vi "Report - Generate Report.vi"(8 "error in":errorcluster, 11 "Fileid":string) -> (0 "error out":errorcluster)   [LabVIEW 2019]
uses:
  Controls/Report - State.ctl
  Controls/Report - Data Structure.ctl
  <vilib>/httpClient/ClientHandle.ctl
  Controls/FGV States.ctl
  Controls/eFGV States.ctl
  Controls/JSON - Fileid.ctl
  Controls/JSON - Report.ctl
  <vilib>/Utility/sysdir.llb/System Directory Type.ctl
  <vilib>/httpClient/POSTBuffer.vi
  <userlib>/_OpenG.lib/array/array.llb/Remove Duplicates from 1D Array (String)__ogtk.vi
  <userlib>/_OpenG.lib/array/array.llb/Delete Elements from 1D Array (String)__ogtk.vi
  <vilib>/Utility/config.llb/Read Key (String).vi
  <vilib>/httpClient/LabVIEWHTTPClient.lvlib
  <vilib>/Utility/config.llb/NI_LVConfig.lvlib
panel:
  in  "Plot":bool
  out "Current stage":T1
  in  "Back":bool
  in  "Forward":bool
  in  "Pages":u32
  out "Total":u32
  out "data":T2(array[cluster])
  in  "Cancel":bool
  in  "Generate":bool
  in  "Search":string
  in  "Listbox":i32(listbox)=-1 caption="Select File to Export"
  # "of"
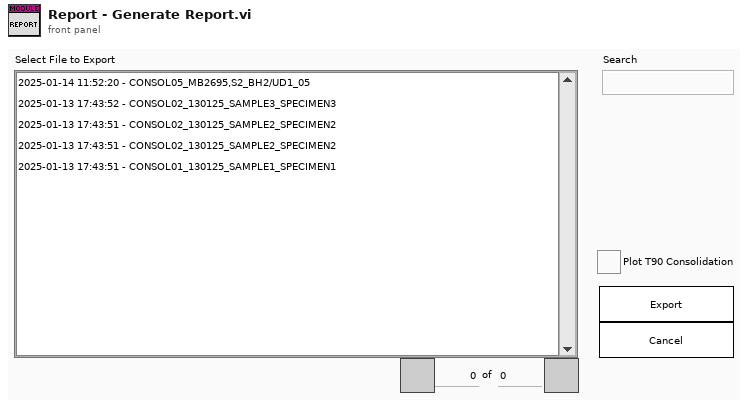
[diagram p1: front panel]
types:
  T1 = typedef "Report - State.ctl" = enum16{"Init", "Get File List", "Get Station Name", "Parse File List", "Idle", "Prepare to Generate", "Get Report", "Parse Report", "Get Data", "View T90", "Parse Data", "Convert to Excel", "Clean Up", "Close"}
  T2 = cluster{"id":string, "created_date":string, "testname":string, "jobno":string, "jobdesc":string, "sampleid":string, "date":string, "specimentno":string, "depth":string, "height":string, "diameter":string, "weight":string, "done":string}[]
  T3 = typedef "eFGV States.ctl" = enum16{"Init", "Read", "Write", "Exit"}
  T4 = typedef "FGV States.ctl" = enum16{"Read", "Write"}
  T5 = typedef "Report - Data Structure.ctl" = cluster{"API Ref":T6, "FileList":string[][], "Fileid":string, "testname":string[], "testtype":string[], "tdms":refnum<k34>, "TDMS Path":path, "tdms_path":string, "excel_path":string, "Excel Path":path, "List Name":string[], "Station Name":string[], "Plot":bool, "Tangent Point":string}
  T6 = typedef "LabVIEWHTTPClient.lvlib/ClientHandle.ctl" = refnum<k1>
  T7 = enum32{"Invalid", "Default", "Floating", "Floating/Auto-Hide", "Modal"}
  T8 = enum32{"Invalid", "Standard", "Closed", "Hidden", "Minimized", "Maximized"}
  T9 = typedef "JSON - Fileid.ctl" = cluster{"status":string, "data":cluster{"id":string, "created_date":string, "testname":string, "jobno":string, "jobdesc":string, "sampleid":string, "date":string, "specimentno":string, "depth":string, "height":string, "diameter":string, "weight":string, "done":string}[]}
  T10 = cluster{"status":string, "data":cluster{"id":string, "created_date":string, "filename":string, "stage":string, "testplan":string, "station":string, "status":string, "delete":string}[]}
  T11 = typedef "JSON - Report.ctl" = cluster{"status":string, "data":cluster{"testname":string, "testtype":string}[]}
  T12 = enum16{"open", "open or create", "create or replace", "create", "open (read-only)"}
  T13 = cluster{"id":string, "created_date":string, "filename":string, "stage":string, "testplan":string, "station":string, "status":string, "delete":string}[]
  T14 = cluster{"id":string, "created_date":string, "filename":string, "stage":string, "testplan":string, "station":string, "status":string, "delete":string}
  T15 = typedef "eventvkey.ctl" = enum16{"ASCII", "Enter", "Return", "Shift", "Ctrl", "Alt", "Cmd", "Opt", "Caps", "NumLock", "Clear", "Break", "Up", "Down", "Left", "Right", "Insert", "Delete", "Home", "End", "PageUp", "PageDown", "Escape", "Help", "Pause", "ScrollLock", "F1", "F2", "F3", "F4", "F5", "F6", "F7", "F8", "F9", "F10", "F11", "F12", "F13", "F14", "F15", "F16", "F17", "F18", "F19", "F20", "F21", "F22", "F23", "F24", "Play", "VolumeUp", "VolumeDown", "Mute", "Two Byte Char"}
  T16 = typedef "System Directory Type.ctl" = i32
  T17 = typedef "NI_LVConfig.lvlib/Config Data RefNum.ctl" = refnum<k1>
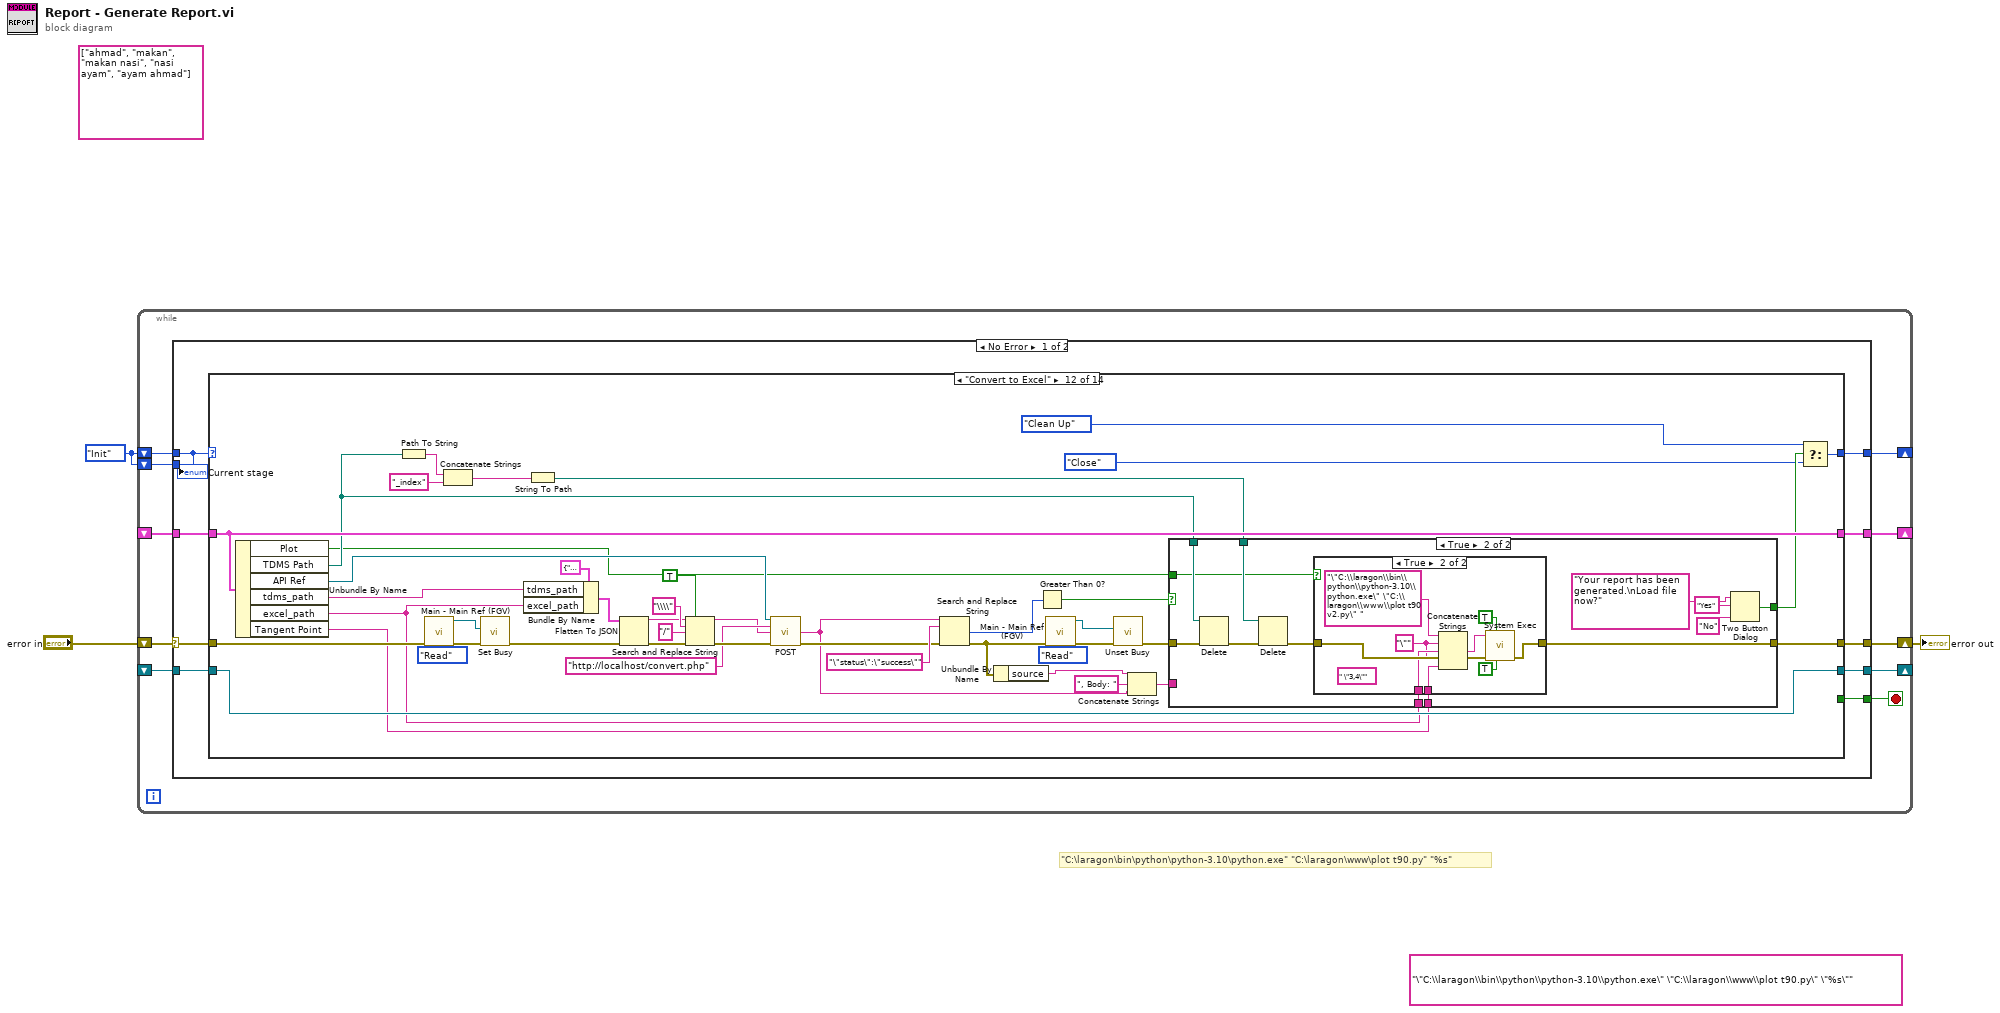
[diagram p0: block diagram]
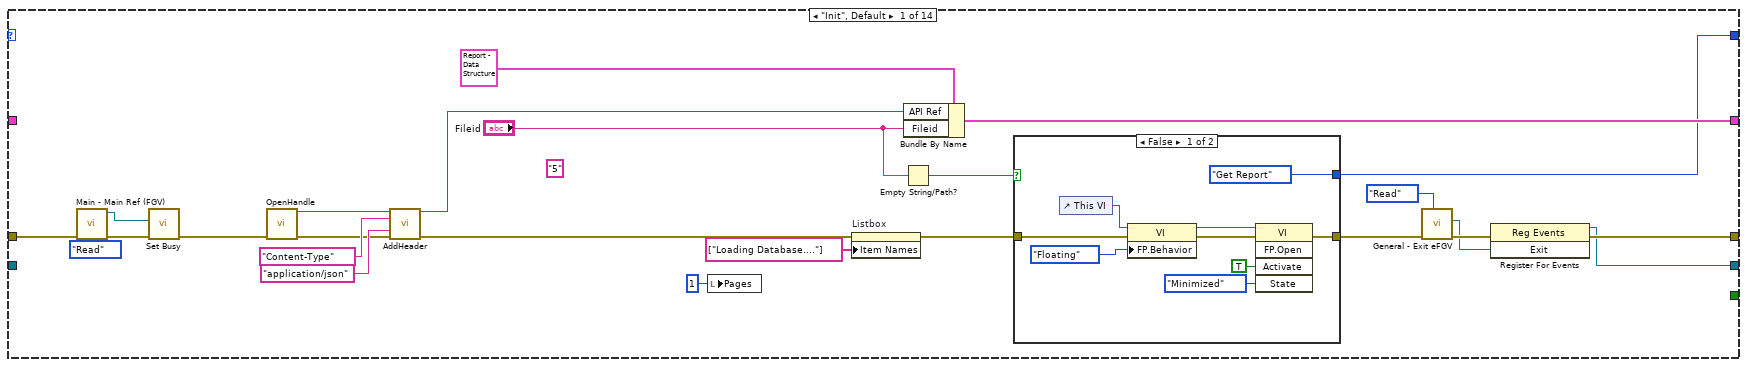
[diagram p2: hidden frame]
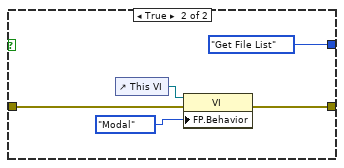
[diagram p3: hidden frame]
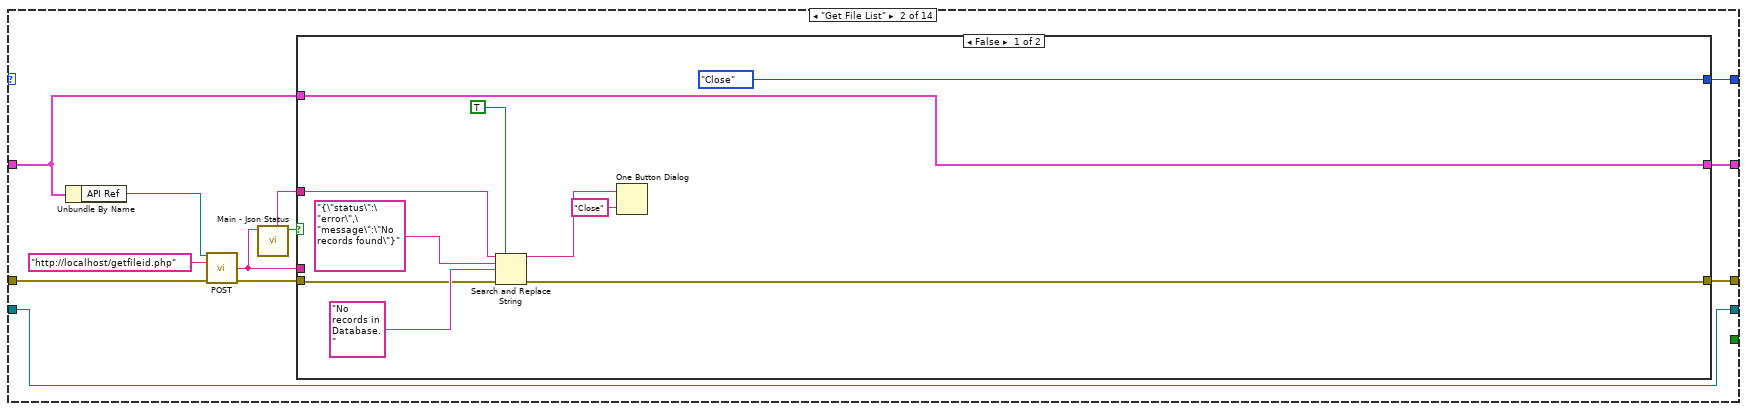
[diagram p4: hidden frame]
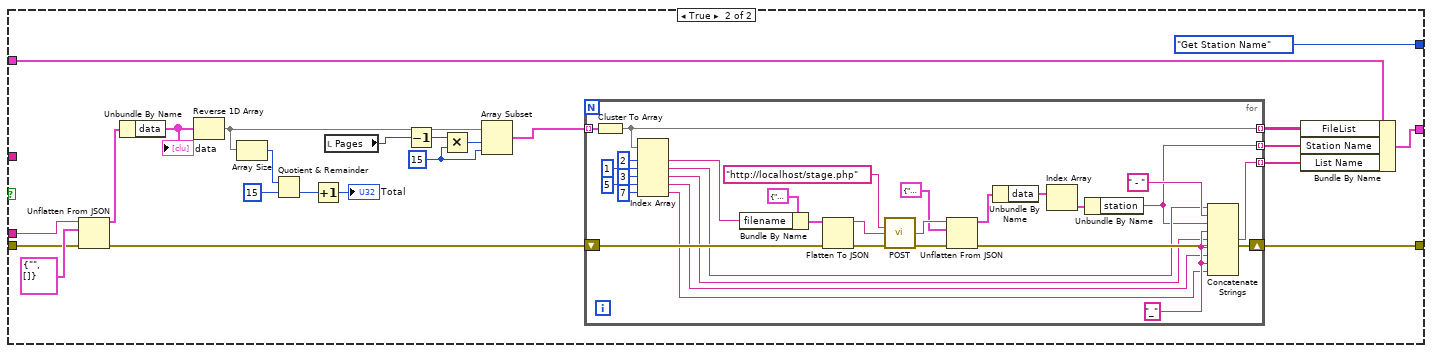
[diagram p5: hidden frame]
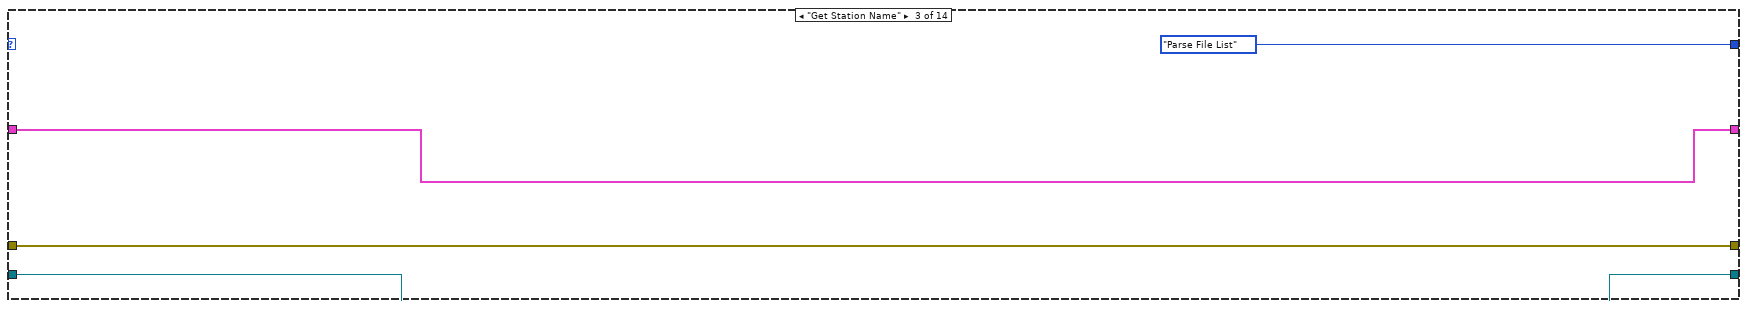
[diagram p6: hidden frame]
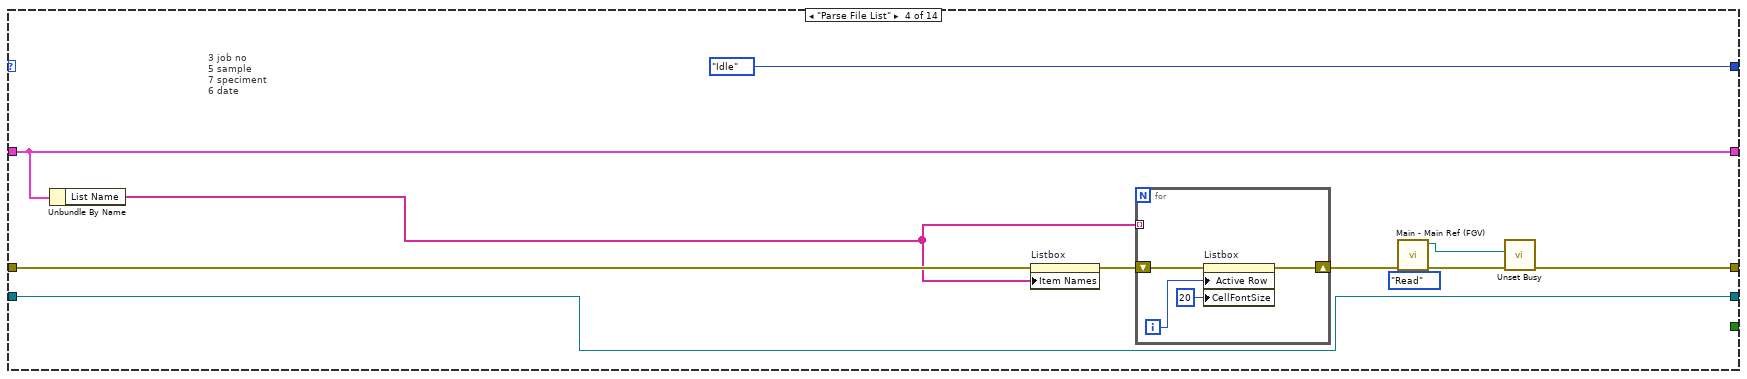
[diagram p7: hidden frame]
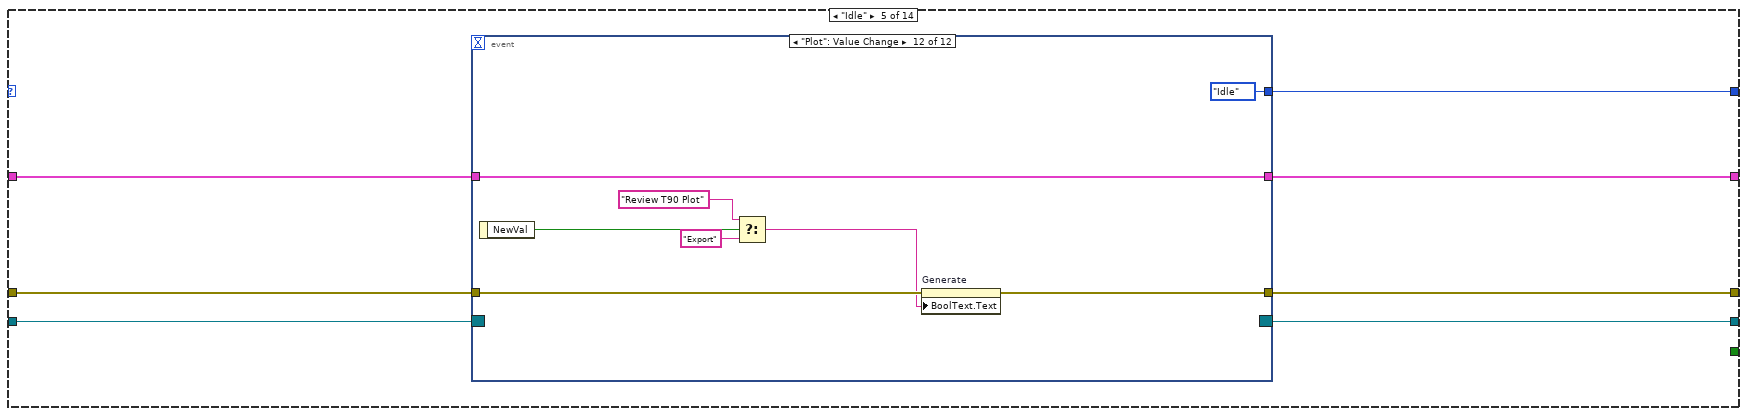
[diagram p8: hidden frame]
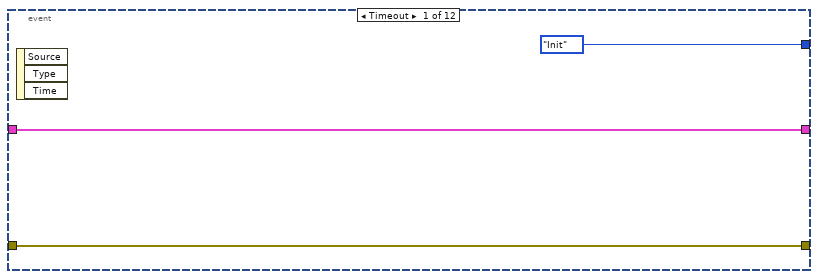
[diagram p9: hidden frame]
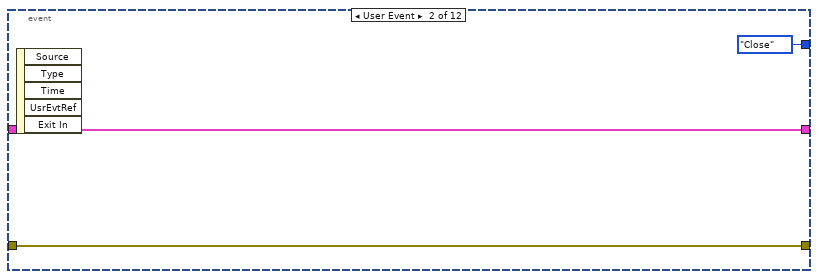
[diagram p10: hidden frame]
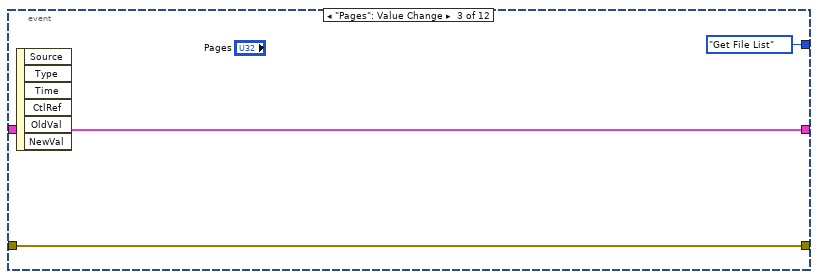
[diagram p11: hidden frame]
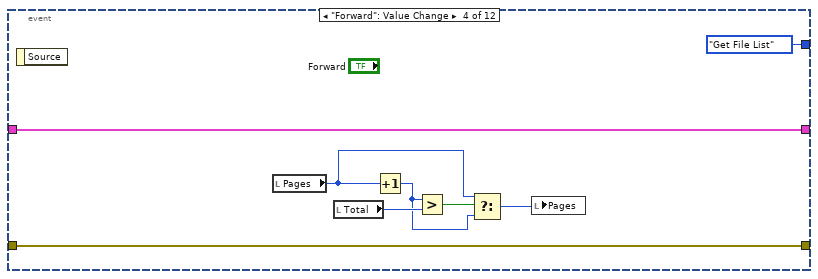
[diagram p12: hidden frame]
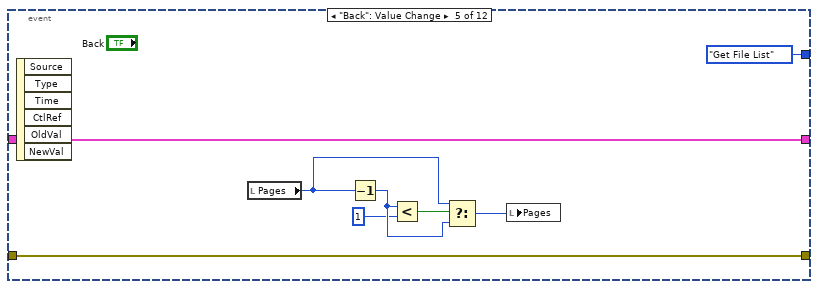
[diagram p13: hidden frame]
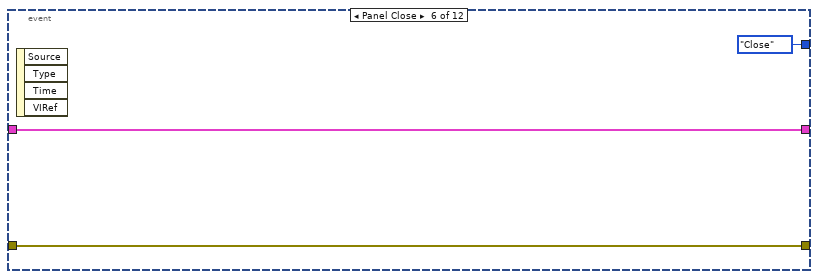
[diagram p14: hidden frame]
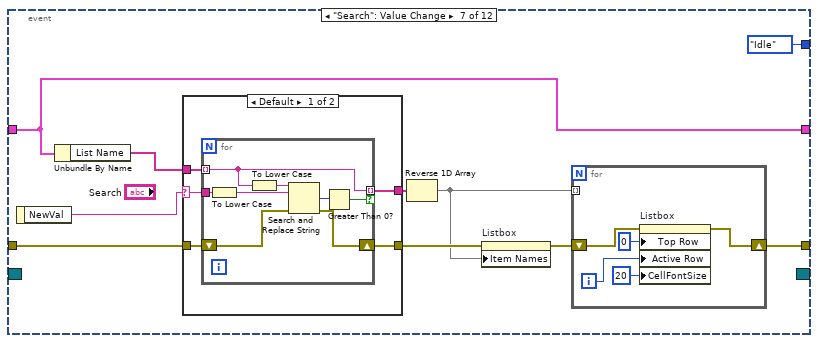
[diagram p15: hidden frame]
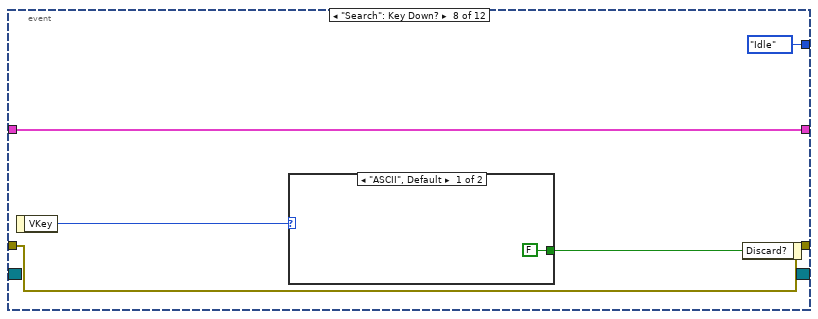
[diagram p17: hidden frame]
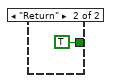
[diagram p18: hidden frame]
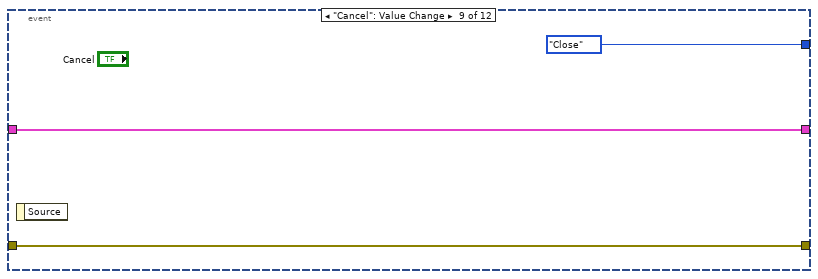
[diagram p19: hidden frame]
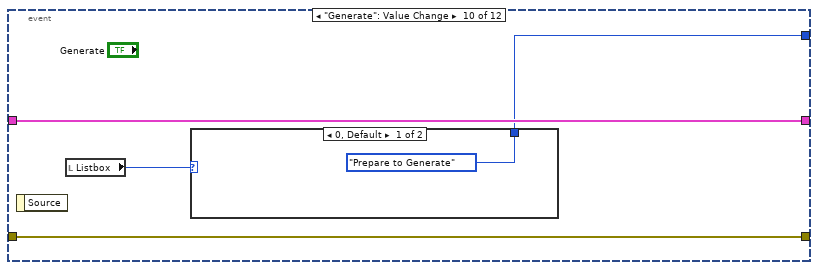
[diagram p20: hidden frame]
diagram:
  (unwired) "\"C:\\laragon\\bin\\python\\python-3.10\\python.exe\" \"C:\\laragon\\www\\plot t90.py\" \"%s\"" ("command line")
  w1 = Report_-_State."Init"
  (unwired) string[] ["ahmad", "makan", "makan nasi", "nasi ayam", "ayam ahmad"]
  # "\"C:\\laragon\\bin\\python\\python-3.10\\python.exe\" \"C:\\laragon\\www\\plot t90.py\" \"%s\""
  n1 = while {
    shift-right: [w10] -> w2
    shift-left: "error in" -> [w13]
    shift-right: [w11] -> _
    shift-left: w1 -> [w12]
    shift-right: [w9] -> _
    shift-left: _ -> [w8]
    shift-left: w1 -> [w6]
    shift-right: [w5] -> _
    shift-left: _ -> [w4]
    stop <- w7 stop-if-true
    n2 = case shown="No Error" w13 {
      selector: w13 -> [w20 w547]
      tunnel: w12 -> [w22 _]
      tunnel: [w21 Report_-_State."Close"] -> w11
      tunnel: [w19 w544] -> w10
      tunnel: [w18 w545] -> w9
      tunnel: w8 -> [w17 w545]
      tunnel: [w16 _] -> w7
      tunnel: w6 -> [_ w538]
      tunnel: [w15 w534] -> w5
      tunnel: w4 -> [w14 w534]
      frame No Error {
        n3 = case shown="\"Convert to Excel\"" w22 {
          tunnel: [w40 w71 Report_-_State."Parse File List" Report_-_State."Idle" w159 Report_-_State."Get Report" w285 Report_-_State."Get Data" w344 Report_-_State."Parse Data" w384 w429 Report_-_State."Close" Report_-_State."Idle"] -> w21
          tunnel: w20 -> [w35 w72 w139 w149 w161 w268 w298 w331 w345 w372 w377 w425 w493 w530]
          tunnel: [w29 w69 w139 w143 w160 w282 w289 w328 w341 w371 w382 w433 w498 w522] -> w19
          tunnel: [w41 w66 w137 w147 w157 w273 w290 w327 w339 w367 w386 w432 w497 T5 {"API Ref"=refnum, "FileList"=[], "Fileid"="", "testname"=[], "testtype"=[], "tdms"=refnum, "TDMS Path"=path "", "tdms_path"="", "excel_path"="", "Excel Path"=path "", "List Name"=[], "Station Name"=[], "Plot"=FALSE, "Tangent Point"=""}] -> w18
          tunnel: w17 -> [_ w67 w137 w147 w158 w272 w292 w330 w338 w366 w389 w432 w497 w529]
          tunnel: [_ _ _ _ _ _ _ _ _ _ _ _ _ TRUE] -> w16
          tunnel: [w27 w62 w136 w140 w155 w265 w284 w323 w340 w373 w374 w413 w484 w521] -> w15
          tunnel: w14 -> [_ w62 w136 w140 w156 w265 w284 w323 w340 w373 w374 w413 w484 w521]
          frame "Init", Default {
            (unwired) "5"
            n4 = call "Main - Main Ref (FGV).vi"("Action"=FGV_States."Read", "error in"=w35) -> ("error out"=w36:errorcluster, "This VI out"=w34:refnum<vi>)  [unwired: 8 in]
            n5 = call <vilib>:"Set Busy.vi"("error in (no error)"=w36, "VI reference (current VI)"=w34) -> ("error out"=w38:errorcluster)  [unwired: 8 in, 1 out]
            n6 = call <vilib>:"OpenHandle.vi"("error in (no error)"=w38) -> ("client handle out"=w45:T6, "error out"=w44:errorcluster)  [unwired: 13 in]
            n7 = call <vilib>:"AddHeader.vi"("client handle"=w45, "header"="Content-Type", "value"="application/json", "error in (no error)"=w44) -> ("client handle out"=w42:T6, "error out"=w26:errorcluster)  [unwired: 10 in]
            n8 = local write "Pages"(u32 1 ("Pages")) -> ()
            n9 = property on="Listbox" class="LstBox (strict)"(error in=w26, "Item Names"=string[] ["Loading Database...."]) -> (error out=w25:errorcluster)  [unwired: 1 in, 1 out]
            n10 = Empty String/Path?(string/path="Fileid") -> (empty?=w39:bool)
            n11 = Bundle By Name(cluster=T5 {"API Ref"=refnum, "FileList"=[], "Fileid"="", "testname"=[], "testtype"=[], "tdms"=refnum, "TDMS Path"=path "", "tdms_path"="", "excel_path"="", "Excel Path"=path "", "List Name"=[], "Station Name"=[], "Plot"=FALSE, "Tangent Point"=""}, "API Ref"=w42, "Fileid"="Fileid") -> (w41:T5)
            n12 = case shown="False" w39 {
              tunnel: [Report_-_State."Get Report" ("f") Report_-_State."Get File List" ("f")] -> w40
              tunnel: w25 -> [w52 w58]
              tunnel: [w50 w57] -> w32
              frame False {
                n13 = control-ref of="This VI"() -> (w49:refnum<vi>)
                n14 = property class="VI"(reference=w49, error in=w52, "FP.Behavior"=T7."Floating" ("Front Panel Window:Behavior")) -> (reference out=w48:refnum<vi>, error out=w51:errorcluster)
                n15 = invoke class="VI" method="FP.Open"(reference=w48, error in=w51, "Activate"=TRUE ("Activate?"), "State"=T8."Minimized") -> (error out=w50:errorcluster)  [unwired: 1 in, 4 out]
              }
              frame True {
                n16 = control-ref of="This VI"() -> (w60:refnum<vi>)
                n17 = property class="VI"(reference=w60, error in=w58, "FP.Behavior"=T7."Modal" ("Front Panel Window:Behavior")) -> (error out=w57:errorcluster)  [unwired: 1 out]
              }
            }
            n18 = call "General - Exit eFGV.vi"("eFGV States"=eFGV_States."Read", "error in (no error)"=w32) -> ("error out"=w31:errorcluster, "Exit"=w28:refnum<user-event>)  [unwired: 7 in, 1 out]
            n19 = register-events(error in=w31, w28) -> (reference out=w27:refnum<event-registration>, error out=w29:errorcluster)  [unwired: 1 in]
          }
          frame "Get File List" {
            n20 = Unbundle By Name(w67) -> ("API Ref"=w68:T6)
            n21 = call-poly <vilib>:"POST.vi"("client handle"=w68, "url"="http://localhost/getfileid.php", "error in (no error)"=w72) -> ("body"=w65:string, "error out"=w70:errorcluster)  [unwired: 9 in, 2 out]
            n22 = call "Main - Json Status.vi"("json"=w65) -> ("Success?"=w64:bool, "message"=w63:string)  [unwired: 9 in]
            n23 = case shown="False" w64 {
              tunnel: [Report_-_State."Close" Report_-_State."Get Station Name"] -> w71
              tunnel: w70 -> [w74 w104]
              tunnel: [w75 w97] -> w69
              tunnel: w65 -> [_ w103]
              tunnel: w67 -> [w82 w100]
              tunnel: [w82 w98] -> w66
              tunnel: w63 -> [w77 _]
              frame False {
                n24 = Search and Replace String(replace all?=TRUE ("replace all? (F)"), input string=w77, search string="{\"status\":\"error\",\"message\":\"No records found\"}", replace string="No records in Database." ("replace string (\"\")"), error in=w74) -> (result string=w78:string, error out=w75:errorcluster)  [unwired: 3 in, 2 out]
                n25 = One Button Dialog(message=w78, button name ("OK")="Close") -> ()  [unwired: 1 out]
              }
              frame True {
                w90 = 15 ("length")
                n26 = Unflatten From JSON(JSON string=w103, type and defaults=T9 {"status"="", "data"=[]}, error in (no error)=w104) -> (value=w101:T9, error out=w85:errorcluster)  [unwired: 4 in]
                n27 = Unbundle By Name(w101) -> ("data"=w102:T2)
                "data" <- w102
                n28 = Reverse 1D Array(array=w102) -> (reversed array=w89:T2)
                n29 = Array Size(array=w89) -> (size(s)=w93:i32)
                n30 = Quotient & Remainder(x=w93, y=15) -> (floor(x/y)=w94:i32)  [unwired: 1 out]
                n31 = Increment(x=w94) -> (x+1=→"Total":i32)
                n32 = local read "Pages"() -> (w86:u32)
                n33 = Decrement(x=w86) -> (x-1=w87:u32)
                n34 = Multiply(x=w87, y=w90) -> (x*y=w91:u32)
                n35 = Array Subset(array=w89, index=w91, length=w90) -> (w88:T2)
                n36 = for {
                  tunnel: w88 -> [w135] mode=indexing
                  tunnel: [w134] -> w99 mode=indexing
                  shift-right: [w114] -> w97
                  shift-left: w85 -> [w115]
                  tunnel: [w108] -> w95 mode=indexing
                  tunnel: [w107] -> w96 mode=indexing
                  w119 = "_" ("string")
                  n37 = Cluster To Array(cluster=w135) -> (array=w134:string[])
                  n38 = Index Array(array=w134, index #1=2 ("disabled index (col)"), index #2=1 ("index (col)"), index #3=3 ("index (col)"), index #4=5 ("index (col)"), index #5=7 ("index (col)")) -> (element #1=w113:string, element #2=w112:string, element #3=w111:string, element #4=w110:string, element #5=w109:string)
                  n39 = Bundle By Name(cluster=cluster{"action":string, "filename":string} {"action"="read", "filename"=""}, "filename"=w113) -> (w124:cluster{"action":string, "filename":string})
                  n40 = Flatten To JSON(anything=w124, error in (no error)=w115) -> (JSON string=w125:string, 11:w128:errorcluster)  [unwired: 1 in]
                  n41 = call-poly <vilib>:"POST.vi"("url"="http://localhost/stage.php", "buffer"=w125, "error in (no error)"=w128) -> ("body"=w126:string, "error out"=w127:errorcluster)  [unwired: 9 in, 2 out]
                  n42 = Unflatten From JSON(JSON string=w126, type and defaults=T10 {"status"="read", "data"=[]} ("Cluster"), error in (no error)=w127) -> (value=w123:T10, error out=w114:errorcluster)  [unwired: 4 in]
                  n43 = Unbundle By Name(w123) -> ("data"=w122:T13)
                  n44 = Index Array(array=w122) -> (element=w121:T14)  [unwired: 1 in]
                  n45 = Unbundle By Name(w121) -> ("station"=w107:string)
                  n46 = Concatenate Strings(w112, " - " ("string"), w107, w119, w111, w119, w110, w119, w109) -> (w108:string)
                }
                n47 = Bundle By Name(cluster=w100, "FileList"=w99, "Station Name"=w96, "List Name"=w95) -> (w98:T5)
              }
            }
          }
          frame "Get Station Name" {
          }
          frame "Parse File List" {
            # "3 job no\n5 sample\n7 speciment\n6 date"
            n48 = Unbundle By Name(w147) -> ("List Name"=w141:string[])
            n49 = property on="Listbox" class="LstBox (strict)"(error in=w149, "Item Names"=w141) -> (error out=w148:errorcluster)  [unwired: 1 in, 1 out]
            n50 = for {
              shift-right: [w152] -> w145
              shift-left: w148 -> [w153]
              tunnel: w141 -> [_] mode=indexing
              i -> [w151]
              n51 = property on="Listbox" class="LstBox (strict)"(error in=w153, "Active Row"=w151, "CellFontSize"=u32 20 ("Active Row:Cell Font:Size")) -> (error out=w152:errorcluster)  [unwired: 1 in, 1 out]
            }
            n52 = call "Main - Main Ref (FGV).vi"("Action"=FGV_States."Read", "error in"=w145) -> ("error out"=w144:errorcluster, "This VI out"=w142:refnum<vi>)  [unwired: 8 in]
            n53 = call <vilib>:"Unset Busy.vi"("error in (no error)"=w144, "VI reference (current VI)"=w142) -> ("error out"=w143:errorcluster)  [unwired: 9 in]
          }
          frame "Idle" {
            n54 = event shown="[11] \"Plot\": Value Change" {
              selector: w156 -> [_ _ _ _ _ _ _ _ _ _ _ _]
              dyn-events: [_ _ _ _ _ _ _ _ _ _ _ _] -> w155
              timeout: _ -> [_ _ _ _ _ _ _ _ _ _ _ _]
              tunnel: w161 -> [w164 w167 w168 w176 w186 w187 w195 w220 w228 w232 w249 w260]
              tunnel: [w164 w167 w168 w176 w186 w187 w194 w220 w228 w232 w246 w261] -> w160
              tunnel: [Report_-_State."Init" Report_-_State."Close" ("f") Report_-_State."Get File List" ("f") Report_-_State."Get File List" ("f") Report_-_State."Get File List" ("f") Report_-_State."Close" Report_-_State."Idle" Report_-_State."Idle" ("f") Report_-_State."Close" w230 w237 Report_-_State."Idle" ("f")] -> w159
              tunnel: w158 -> [w162 w166 w170 w177 w185 w188 w192 w224 w229 w233 w252 w263]
              tunnel: [w162 w166 w170 w177 w185 w188 w192 w224 w229 w233 w252 w263] -> w157
              event Timeout {
                n55 = event-data() -> ()  [unwired: 1 in, 3 out]
              }
              event User Event {
                n56 = event-data() -> ()  [unwired: 1 in, 5 out]
              }
              event "Pages": Value Change {
                n57 = event-data() -> ()  [unwired: 1 in, 6 out]
              }
              event "Forward": Value Change {
                n58 = event-data() -> ()  [unwired: 1 in, 1 out]
                n59 = local read "Pages"() -> (w173:u32)
                n60 = local read "Total"() -> (w175:u32)
                n61 = Increment(x=w173) -> (x+1=w172:u32)
                n62 = Greater?(x=w172, y=w175) -> (0:w174:bool)
                n63 = Select(t=w173, s=w174, f=w172) -> (s? t:f=w171:u32)
                n64 = local write "Pages"(w171) -> ()
              }
              event "Back": Value Change {
                n65 = event-data() -> ()  [unwired: 1 in, 6 out]
                n66 = local read "Pages"() -> (w182:u32)
                n67 = Decrement(x=w182) -> (x-1=w181:u32)
                n68 = Less?(x=w181, y=u32 1) -> (x < y?=w183:bool)
                n69 = Select(t=w182, s=w183, f=w181) -> (s? t:f=w180:u32)
                n70 = local write "Pages"(w180) -> ()
              }
              event Panel Close {
                n71 = event-data() -> ()  [unwired: 1 in, 4 out]
              }
              event "Search": Value Change {
                n72 = event-data() -> ("NewVal"=w193:string)  [unwired: 1 in]
                n73 = Unbundle By Name(w192) -> ("List Name"=w190:string[])
                n74 = case shown="Default" w193 {
                  selector: w193 -> [w205 _]
                  tunnel: w190 -> [w209 w219]
                  tunnel: w195 -> [w208 w218]
                  tunnel: [w207 w218] -> w198
                  tunnel: [w206 w219] -> w196
                  frame Default {
                    n75 = for {
                      tunnel: w205 -> [w217]
                      tunnel: [w214] -> w206 mode=indexing if=w215
                      tunnel: w209 -> [w214] mode=indexing
                      shift-right: [w212] -> w207
                      shift-left: w208 -> [w213]
                      n76 = To Lower Case(string=w217) -> (all lower case string=w211:string)
                      n77 = To Lower Case(string=w214) -> (all lower case string=w210:string)
                      n78 = Search and Replace String(input string=w210, search string=w211, error in=w213) -> (number of replacements=w216:i32, error out=w212:errorcluster)  [unwired: 5 in, 2 out]
                      n79 = Greater Than 0?(x=w216) -> (x > 0?=w215:bool)
                    }
                  }
                  frame "" {
                  }
                }
                n80 = Reverse 1D Array(array=w196) -> (reversed array=w191:string[])
                n81 = property on="Listbox" class="LstBox (strict)"(error in=w198, "Item Names"=w191) -> (error out=w197:errorcluster)  [unwired: 1 in, 1 out]
                n82 = for {
                  shift-right: [w202] -> w194
                  shift-left: w197 -> [w203]
                  tunnel: w191 -> [_] mode=indexing
                  i -> [w201]
                  n83 = property on="Listbox" class="LstBox (strict)"(error in=w203, "Top Row"=0, "Active Row"=w201, "CellFontSize"=u32 20 ("Active Row:Cell Font:Size")) -> (error out=w202:errorcluster)  [unwired: 1 in, 1 out]
                }
              }
              event "Search": Key Down? {
                n84 = event-data() -> ("VKey"=w222:T15)  [unwired: 1 in]
                n85 = case shown="\"ASCII\", Default" w222 {
                  tunnel: [FALSE TRUE] -> w221
                  frame "ASCII", Default {
                  }
                  frame "Return" {
                  }
                }
                n86 = event-data("Discard?"=w221) -> ()  [unwired: 1 in, 1 out]
              }
              event "Cancel": Value Change {
                n87 = event-data() -> ()  [unwired: 1 in, 1 out]
              }
              event "Generate": Value Change {
                n88 = event-data() -> ()  [unwired: 1 in, 1 out]
                n89 = local read "Listbox"() -> (w231:i32)
                n90 = case shown="0, Default" w231 {
                  tunnel: [Report_-_State."Prepare to Generate" Report_-_State."Idle"] -> w230
                  frame 0, Default {
                  }
                  frame -1 {
                    n91 = One Button Dialog(message="Please select a file") -> ()  [unwired: 1 in, 1 out]
                  }
                }
              }
              event "Listbox": Double Click {
                n92 = event-data() -> ("Row"=w247:i32)  [unwired: 1 in]
                n93 = property on="Listbox" class="LstBox (strict)"(error in=w249) -> (error out=w250:errorcluster, "Item Names"=w248:string[])  [unwired: 1 in, 1 out]
                n94 = Index Array(array=w248, index=w247) -> (element=w245:string)
                n95 = Format Into String(format string="Generate report %s?" ("message"), initial string="", error in=w250, w245) -> (resulting string=w242:string, error out=w246:errorcluster)
                n96 = Two Button Dialog(message=w242, 2:"Yes" ("T button name (\"OK\")")) -> (T button?=w238:bool)  [unwired: 1 in]
                n97 = local read "Listbox"() -> (w251:i32)
                n98 = case shown="0, Default" w251 {
                  tunnel: [Report_-_State."Prepare to Generate" Report_-_State."Idle"] -> w240
                  frame 0, Default {
                  }
                  frame -1 {
                    n99 = One Button Dialog(message="Please select a file") -> ()  [unwired: 1 in, 1 out]
                  }
                }
                n100 = Select(t=w240, s=w238, f=Report_-_State."Idle") -> (s? t:f=w237:T1)
              }
              event "Plot": Value Change {
                n101 = event-data() -> ("NewVal"=w258:bool)  [unwired: 1 in]
                n102 = Select(t="Review T90 Plot" ("Boolean Text.Text"), s=w258, f="Export") -> (s? t:f=w256:string)
                n103 = property on="Generate" class="Bool"(error in=w260, "BoolText.Text"=w256) -> (error out=w261:errorcluster)  [unwired: 1 in, 1 out]
              }
            }
          }
          frame "Prepare to Generate" {
            n104 = call "Main - Main Ref (FGV).vi"("Action"=FGV_States."Read", "error in"=w268) -> ("error out"=w269:errorcluster, "This VI out"=w267:refnum<vi>)  [unwired: 8 in]
            n105 = call <vilib>:"Set Busy.vi"("error in (no error)"=w269, "VI reference (current VI)"=w267) -> ("error out"=w271:errorcluster)  [unwired: 8 in, 1 out]
            n106 = property on="Listbox" class="LstBox (strict)"(error in=w271) -> (error out=w282:errorcluster, "Item Names"=w280:string[])  [unwired: 1 in, 1 out]
            n107 = Unbundle By Name(w272) -> ("FileList"=w279:string[][], "List Name"=w266:string[])
            n108 = Index Array(array=w279, index (col)=0 ("disabled index (col)")) -> (element=w276:string[])  [unwired: 1 in]
            n109 = Index Array(array=w280, index="Listbox") -> (element=w277:string)
            n110 = Search 1D Array(1D array=w266, element=w277) -> (index of element=w275:i32)  [unwired: 1 in]
            n111 = Index Array(array=w276, index=w275) -> (element=w274:string)
            n112 = Bundle By Name(cluster=w272, "Plot"="Plot", "Fileid"=w274) -> (w273:T5)
          }
          frame "Get Report" {
            n113 = Unbundle By Name(w292) -> ("API Ref"=w291:T6, "Fileid"=w297:string)
            n114 = Bundle By Name(cluster=cluster{"fileid":string} {"fileid"=""}, "fileid"=w297) -> (w299:cluster{"fileid":string})
            n115 = Flatten To JSON(anything=w299, error in (no error)=w298) -> (JSON string=w294:string, 11:w295:errorcluster)  [unwired: 1 in]
            n116 = call-poly <vilib>:"POST.vi"("client handle"=w291, "url"="http://localhost/report.php", "buffer"=w294, "error in (no error)"=w295) -> ("body"=w288:string, "error out"=w293:errorcluster)  [unwired: 8 in, 2 out]
            n117 = call "Main - Json Status.vi"("json"=w288) -> ("Success?"=w287:bool, "message"=w286:string)  [unwired: 9 in]
            n118 = case shown="True" w287 {
              tunnel: w293 -> [w302 w318]
              tunnel: w292 -> [w305 w312]
              tunnel: [w305 w309] -> w290
              tunnel: [w301 w308] -> w289
              tunnel: w288 -> [_ w307]
              tunnel: w286 -> [w304 _]
              tunnel: [Report_-_State."Close" Report_-_State."Parse Report"] -> w285
              frame False {
                n119 = One Button Dialog(message=w304) -> ()  [unwired: 1 in, 1 out]
                n120 = call <vilib>:"Clear Errors.vi"("error in (no error)"=w302) -> ("error out"=w301:errorcluster)  [unwired: 5 in, 1 out]
              }
              frame True {
                n121 = Unflatten From JSON(JSON string=w307, type and defaults=T11 {"status"="", "data"=[]}, error in (no error)=w318) -> (value=w316:T11, error out=w308:errorcluster)  [unwired: 4 in]
                n122 = Unbundle By Name(w316) -> ("data"=w317:cluster{"testname":string, "testtype":string}[])
                n123 = for {
                  tunnel: w317 -> [w322] mode=indexing
                  tunnel: [w321] -> w313 mode=indexing
                  tunnel: [w320] -> w314 mode=indexing
                  n124 = Unbundle By Name(w322) -> ("testtype"=w321:string, "testname"=w320:string)
                }
                n125 = call-poly <userlib>:"Remove Duplicates from 1D Array__ogtk.vi"("Input Array"=w314) -> ("Output Array"=w310:string[], "indices of removed elements"=w315:i32[])
                n126 = call-poly <userlib>:"Delete Elements from Array__ogtk.vi"("indices"=w315, "array"=w313) -> ("array w/ subset deleted"=w311:string[])  [unwired: 8 in, 1 out]
                n127 = Bundle By Name(cluster=w312, "testtype"=w311, "testname"=w310) -> (w309:T5)
              }
            }
          }
          frame "Parse Report" {
            n128 = Format Date/Time String(time format string (%c)="%H%M%S") -> (date/time string=w334:string)  [unwired: 2 in]
            n129 = Concatenate Strings("convert-" ("string"), w334, ".tdms" ("string")) -> (w332:string)
            n130 = Temporary Directory() -> (w324:path)
            n131 = Build Path(base path=w324, name or relative path=w332) -> (appended path=w325:path)
            n132 = TDMS Open(8:w331, 10:T12."create" ("operation (0:open)"), 11:w325) -> (0:w328:errorcluster, 3:w329:refnum<k34>)  [unwired: 4 in]
            n133 = Bundle By Name(cluster=w330, "TDMS Path"=w325, "tdms"=w329) -> (w327:T5)
          }
          frame "Get Data" {
            n134 = call "Report - Parse Data to TDMS (SubVI).vi"("error in (no error)"=w345, "Cluster"=w338) -> ("error out"=w342:errorcluster, "Cancel?"=w343:bool)  [unwired: 8 in]
            n135 = case shown="False" w343 {
              tunnel: [w350 Report_-_State."Idle"] -> w344
              tunnel: w342 -> [w348 w361]
              tunnel: [w349 w360] -> w341
              tunnel: [w347 w359] -> w339
              tunnel: w338 -> [w347 w359]
              frame False {
                n136 = Unbundle By Name(w347) -> ("Plot"=w346:bool)
                n137 = case shown="False" w346 {
                  tunnel: [Report_-_State."Parse Data" Report_-_State."View T90"] -> w350
                  tunnel: [w352 w354] -> w349
                  tunnel: w348 -> [w352 w353]
                  frame False {
                  }
                  frame True {
                    n138 = call "Main - Main Ref (FGV).vi"("Action"=FGV_States."Read", "error in"=w353) -> ("error out"=w356:errorcluster, "This VI out"=w355:refnum<vi>)  [unwired: 8 in]
                    n139 = call <vilib>:"Unset Busy.vi"("error in (no error)"=w356, "VI reference (current VI)"=w355) -> ("error out"=w354:errorcluster)  [unwired: 9 in]
                  }
                }
              }
              frame True {
                n140 = call "Main - Main Ref (FGV).vi"("Action"=FGV_States."Read", "error in"=w361) -> ("error out"=w363:errorcluster, "This VI out"=w362:refnum<vi>)  [unwired: 8 in]
                n141 = call <vilib>:"Unset Busy.vi"("error in (no error)"=w363, "VI reference (current VI)"=w362) -> ("error out"=w360:errorcluster)  [unwired: 9 in]
              }
            }
          }
          frame "View T90" {
            n142 = Unbundle By Name(w366) -> ("Fileid"=w369:string)
            n143 = call "Run Test - T90 Plot (SubVI).vi"("error in (no error)"=w372, "fileid"=w369) -> ("error out"=w371:errorcluster, "Tengent Point"=w368:string)  [unwired: 8 in]
            n144 = Bundle By Name(cluster=w366, "Tangent Point"=w368) -> (w367:T5)
          }
          frame "Parse Data" {
            w393 = T16 1 items=["User Home"=0, "User Desktop"=1, "User Documents"=2, "User Application Data"=3, "User Preferences"=4, "User Temporary"=5, "Public Documents"=6, "Public Application Data"=7, "Public Preferences"=8, "Public Cache"=13, "System Core Libraries"=9, "System Installed Libraries"=10, "Application Files"=11, "Boot Volume Root"=12] ("system directory type")
            n145 = Unbundle By Name(w389) -> ("TDMS Path"=w390:path)
            n146 = call "Main - Main Ref (FGV).vi"("Action"=FGV_States."Read", "error in"=w377) -> ("error out"=w378:errorcluster, "This VI out"=w375:refnum<vi>)  [unwired: 8 in]
            n147 = call <vilib>:"Unset Busy.vi"("error in (no error)"=w378, "VI reference (current VI)"=w375) -> ("error out"=w376:errorcluster)  [unwired: 9 in]
            n148 = call <vilib>:"Get System Directory.vi"("system directory type"=w393) -> ("system directory"=w385:path)  [unwired: 10 in]
            n149 = call "File Dialog"("start path"=w385, "error in"=w376, "pattern (all files)"="*.xlsx", "pattern label"=".xlsx") -> ("selected path"=w380:path, "cancelled"=w383:bool, "error out"=w381:errorcluster)  [unwired: 8 in, 1 out]
            n150 = Path To String(path=w390) -> (string=w388:string)
            n151 = Path To String(path=w380) -> (string=w387:string)
            n152 = case shown="False" w383 {
              tunnel: w389 -> [w400 _]
              tunnel: w388 -> [w399 _]
              tunnel: w387 -> [w398 _]
              tunnel: [w397 T5 {"API Ref"=refnum, "FileList"=[], "Fileid"="", "testname"=[], "testtype"=[], "tdms"=refnum, "TDMS Path"=path "", "tdms_path"="", "excel_path"="", "Excel Path"=path "", "List Name"=[], "Station Name"=[], "Plot"=FALSE, "Tangent Point"=""}] -> w386
              tunnel: [Report_-_State."Convert to Excel" Report_-_State."Close"] -> w384
              tunnel: [w395 w401] -> w382
              tunnel: w381 -> [w395 w402]
              tunnel: w380 -> [w394 _]
              frame False {
                n153 = Bundle By Name(cluster=w400, "tdms_path"=w399, "excel_path"=w398, "Excel Path"=w394) -> (w397:T5)
              }
              frame True {
                n154 = call <vilib>:"Clear Errors.vi"("error in (no error)"=w402) -> ("error out"=w401:errorcluster)  [unwired: 5 in, 1 out]
              }
            }
          }
          frame "Convert to Excel" {
            n155 = Unbundle By Name(w432) -> ("Plot"=w406:bool, "TDMS Path"=w418:path, "API Ref"=w438:T6, "tdms_path"=w443:string, "excel_path"=w407:string, "Tangent Point"=w405:string)
            n156 = Path To String(path=w418) -> (string=w417:string)
            n157 = call "Main - Main Ref (FGV).vi"("Action"=FGV_States."Read", "error in"=w425) -> ("error out"=w426:errorcluster, "This VI out"=w423:refnum<vi>)  [unwired: 8 in]
            n158 = Concatenate Strings(w417, "_index" ("string")) -> (w415:string)
            n159 = call <vilib>:"Set Busy.vi"("error in (no error)"=w426, "VI reference (current VI)"=w423) -> ("error out"=w424:errorcluster)  [unwired: 8 in, 1 out]
            n160 = Bundle By Name(cluster=cluster{"tdms_path":string, "excel_path":string} {"tdms_path"="", "excel_path"=""}, "tdms_path"=w443, "excel_path"=w407) -> (w448:cluster{"tdms_path":string, "excel_path":string})
            n161 = String To Path(string=w415) -> (path=w414:path)
            n162 = Flatten To JSON(anything=w448, error in (no error)=w424) -> (JSON string=w445:string, 11:w442:errorcluster)  [unwired: 1 in]
            n163 = Search and Replace String(replace all?=TRUE ("replace all? (F)"), input string=w445, search string="\\\\", replace string="/" ("replace string (\"\")"), error in=w442) -> (result string=w439:string, error out=w441:errorcluster)  [unwired: 3 in, 2 out]
            n164 = call-poly <vilib>:"POST.vi"("client handle"=w438, "url"="http://localhost/convert.php", "buffer"=w439, "error in (no error)"=w441) -> ("body"=w411:string, "error out"=w434:errorcluster)  [unwired: 8 in, 2 out]
            n165 = Search and Replace String(input string=w411, search string="\"status\":\"success\"", error in=w434) -> (number of replacements=w436:i32, error out=w409:errorcluster)  [unwired: 5 in, 2 out]
            n166 = Unbundle By Name(w409) -> ("source"=w408:string)
            n167 = Greater Than 0?(x=w436) -> (x > 0?=w435:bool)
            n168 = call "Main - Main Ref (FGV).vi"("Action"=FGV_States."Read", "error in"=w409) -> ("error out"=w421:errorcluster, "This VI out"=w419:refnum<vi>)  [unwired: 8 in]
            n169 = call <vilib>:"Unset Busy.vi"("error in (no error)"=w421, "VI reference (current VI)"=w419) -> ("error out"=w420:errorcluster)  [unwired: 9 in]
            n170 = Concatenate Strings(w408, ", Body: " ("string"), w411) -> (w410:string)
            n171 = case shown="True" w435 {
              tunnel: w418 -> [_ w470]
              tunnel: w420 -> [w454 w469]
              tunnel: [w455 w461] -> w433
              tunnel: [FALSE ("T button?") w465] -> w431
              tunnel: w414 -> [_ w463]
              tunnel: w410 -> [w450 _]
              tunnel: w407 -> [_ w460]
              tunnel: w406 -> [_ w459]
              tunnel: w405 -> [_ w458]
              frame False {
                n172 = Format Into String(format string="There is an error to generate your report.\n\n%s" ("message"), initial string="", error in=w454, w450) -> (resulting string=w452:string, error out=w455:errorcluster)
                n173 = One Button Dialog(message=w452, button name ("OK")="Close") -> ()  [unwired: 1 out]
              }
              frame True {
                n174 = Delete(path (use dialog)=w470, error in=w469) -> (error out=w464:errorcluster)  [unwired: 3 in, 2 out]
                n175 = Delete(path (use dialog)=w463, error in=w464) -> (error out=w462:errorcluster)  [unwired: 3 in, 2 out]
                n176 = case shown="True" w459 {
                  tunnel: w462 -> [w471 w477]
                  tunnel: [w471 w478] -> w461
                  tunnel: w460 -> [_ w475]
                  tunnel: w458 -> [_ w472]
                  frame False {
                  }
                  frame True {
                    (unwired) " \"3,4\"" ("string")
                    w474 = "\"" ("string")
                    n177 = Concatenate Strings("\"C:\\laragon\\bin\\python\\python-3.10\\python.exe\" \"C:\\laragon\\www\\plot t90 v2.py\" " ("command line"), w474, w475, w474, w472) -> (w473:string)
                    n178 = call <vilib>:"System Exec.vi"("run minimized? (F)"=TRUE, "wait until completion? (T)"=TRUE, "error in (no error)"=w477, "command line"=w473) -> ("error out"=w478:errorcluster)  [unwired: 4 in, 3 out]
                  }
                }
                n179 = Two Button Dialog(message="Your report has been generated.\nLoad file now?", 1:"No" ("F button name (\"Cancel\")"), 2:"Yes" ("T button name (\"OK\")")) -> (T button?=w465:bool)
              }
            }
            n180 = Select(t=Report_-_State."Clean Up", s=w431, f=Report_-_State."Close") -> (s? t:f=w429:T1)
          }
          frame "Clean Up" {
            (unwired) path "C:/Program Files/Microsoft Office/root/Office16/EXCEL.EXE"
            # "- Consolidation report.xlsx"
            n181 = Unbundle By Name(w497) -> ("Plot"=w481:bool, "Excel Path"=w483:path)
            n182 = case shown="False" w481 {
              tunnel: w483 -> [w500 w508]
              tunnel: [w500 w501] -> w482
              frame False {
              }
              frame True {
                n183 = Strip Path(path=w508) -> (stripped path=w503:path, name=w507:string)
                n184 = Match Pattern(string=w507, regular expression=".xlsx") -> (before substring=w505:string)  [unwired: 1 in, 3 out]
                n185 = Concatenate Strings(w505, " - Consolidation report.xlsx" ("regular expression")) -> (w502:string)
                n186 = Build Path(base path=w503, name or relative path=w502) -> (appended path=w501:path)
              }
            }
            n187 = call <vilib>:"Application Directory.vi"() -> ("Application Directory"=w496:path)
            n188 = Build Path(base path=w496, name or relative path="Data\\.env") -> (appended path=w494:path)
            n189 = call <vilib>:"Open Config Data.vi"("error in (no error)"=w493, "configuration file path"=w494) -> ("error out"=w492:errorcluster, "refnum"=w491:T17)  [unwired: 7 in, 1 out]
            n190 = call-poly <vilib>:"Read Key.vi"("section"="Excel" ("key"), "error in (no error)"=w492, "key"="Path" ("default value"), "refnum"=w491) -> ("error out"=w490:errorcluster, "value"=w485:string, "refnum out"=w489:T17)  [unwired: 4 in, 1 out]
            n191 = call <vilib>:"Close Config Data.vi"("error in (no error)"=w490, "refnum"=w489) -> ("error out"=w488:errorcluster)  [unwired: 8 in, 1 out]
            n192 = case shown="Default" w485 {
              tunnel: [w512 w519] -> w498
              tunnel: w482 -> [w511 _]
              tunnel: w485 -> [w510 _]
              tunnel: w488 -> [w509 w519]
              frame Default {
                n193 = Format Into String(format string="\"%s\" \"%s\"" ("command line"), error in=w509, w510, w511) -> (resulting string=w514:string, error out=w513:errorcluster)  [unwired: 1 in]
                n194 = call <vilib>:"System Exec.vi"("run minimized? (F)"=TRUE, "wait until completion? (T)"=FALSE, "error in (no error)"=w513, "command line"=w514) -> ("error out"=w512:errorcluster)  [unwired: 4 in, 3 out]
              }
              frame "" {
                n195 = One Button Dialog(message="Please set excel path in .env file") -> ()  [unwired: 1 in, 1 out]
              }
            }
          }
          frame "Close" {
            n196 = Unbundle By Name(w529) -> ("API Ref"=w528:T6)
            n197 = call <vilib>:"CloseHandle.vi"("client handle"=w528, "error in (no error)"=w530) -> ("error out"=w524:errorcluster)  [unwired: 13 in]
            n198 = call "Main - Main Ref (FGV).vi"("Action"=FGV_States."Read", "error in"=w524) -> ("error out"=w526:errorcluster, "This VI out"=w525:refnum<vi>)  [unwired: 8 in]
            n199 = call <vilib>:"Unset Busy.vi"("error in (no error)"=w526, "VI reference (current VI)"=w525) -> ("error out"=w523:errorcluster)  [unwired: 9 in]
            n200 = control-ref of="This VI"() -> (w520:refnum<vi>)
            n201 = invoke class="VI" method="FP.Close"(reference=w520, error in=w523) -> (error out=w522:errorcluster)  [unwired: 1 in, 2 out]
          }
        }
        "Current stage" <- w22
      }
      frame Error {
        n202 = Unbundle By Name(w547) -> ("source"=w541:string)
        n203 = call <vilib>:"Clear Errors.vi"("error in (no error)"=w547) -> ("error out"=w540:errorcluster)  [unwired: 5 in, 1 out]
        n204 = Format Into String(error in=w540, w538) -> (resulting string=w535:string, error out=w539:errorcluster)  [unwired: 2 in]
        n205 = Concatenate Strings(w541, "\n" ("string"), w535) -> (w537:string)
        n206 = call "Main - Main Ref (FGV).vi"("Action"=FGV_States."Read", "error in"=w539) -> ("error out"=w549:errorcluster, "This VI out"=w548:refnum<vi>)  [unwired: 8 in]
        n207 = call <vilib>:"Unset Busy.vi"("error in (no error)"=w549, "VI reference (current VI)"=w548) -> ("error out"=w546:errorcluster)  [unwired: 9 in]
        n208 = flat-sequence {
          tunnel: w537 -> [w554]
          tunnel: [w553] -> w543
          tunnel: w546 -> [w553]
          frame #0 {
            n209 = One Button Dialog(message=w554) -> ()  [unwired: 1 in, 1 out]
          }
        }
        n210 = Unbundle By Name(w545) -> ("API Ref"=w542:T6)
        n211 = call <vilib>:"CloseHandle.vi"("client handle"=w542, "error in (no error)"=w543) -> ("error out"=w544:errorcluster)  [unwired: 13 in]
        n212 = Wait (ms)(milliseconds to wait=u32 1000) -> ()  [unwired: 1 out]
      }
    }
  }
  "error out" <- w2
